vi "PLC_CODMn 停止命令.vi"   [LabVIEW 2016, in "质控单元V1.lvlib"]
types:
  T1 = cluster{"命令":string, "测量模式":enum16{"水样测量", "标样核查", "零点核查", "跨度核查", "空白测试", "加标回收", "平行样", "校零", "校标"}, "CODMn量程切换":enum32{"H", "L", "AUTO"}}
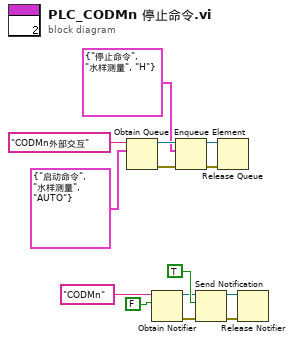
[diagram p0: block diagram]
diagram:
  n1 = Obtain Queue(name (unnamed)="CODMn外部交互" ("名称（未命名）"), element data type=T1 {"命令"="启动命令", "测量模式"=enum."水样测量", "CODMn量程切换"=enum."AUTO"} ("元素")) -> (queue out=w10:refnum<queue>, error out=w9:errorcluster)  [unwired: 3 in, 1 out]
  n2 = Obtain Notifier(name (unnamed)="CODMn" ("名称（未命名）"), notification data type=FALSE) -> (notifier out=w2:refnum<notifier>, error out=w1:errorcluster)  [unwired: 2 in, 1 out]
  n3 = Enqueue Element(queue=w10, element=T1 {"命令"="停止命令", "测量模式"=enum."水样测量", "CODMn量程切换"=enum."H"} ("元素"), error in (no error)=w9) -> (queue out=w12:refnum<queue>, error out=w11:errorcluster)  [unwired: 1 in, 1 out]
  n4 = Send Notification(notification=TRUE ("通知"), notifier=w2, error in (no error)=w1) -> (notifier out=w4:refnum<notifier>, error out=w3:errorcluster)
  n5 = Release Queue(queue=w12, error in (no error)=w11) -> ()  [unwired: 1 in, 3 out]
  n6 = Release Notifier(notifier=w4, error in (no error)=w3) -> ()  [unwired: 1 in, 3 out]
